vi "CheezyAcos.vi"(1 "arg":dbl) -> (0 "acos(arg)":dbl)   [LabVIEW 2016]
uses:
  <userlib>/836-Libraries/Math/CheezyMath/MathConstantsNames.ctl
panel:
  out "Time to run":dbl
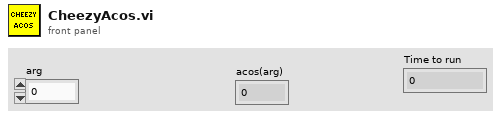
[diagram p1: front panel]
types:
  T1 = typedef "MathConstantsNames.ctl" = enum16{"sq2p1", "sq2m1", "p4", "p3", "p2", "p1", "p0", "q4", "q3", "q2", "q1", "q0", "PIO2"}
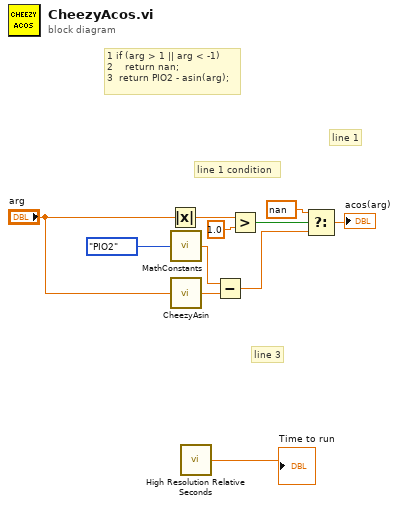
[diagram p0: block diagram]
diagram:
  # "line 3"
  # "line 1"
  # "line 1 condition"
  # "1 if (arg > 1 || arg < -1) \n2    return nan;\n3  return PIO2 - asin(arg);"
  n1 = Absolute Value(x="arg") -> (abs(x)=w11:dbl)
  n2 = call <userlib>:"MathConstants.vi"("Constant Name"=MathConstantsNames."PIO2") -> ("Constant Value"=w5:dbl)
  n3 = call <userlib>:"CheezyAsin.vi"("arg"="arg") -> ("asin(arg)"=w4:dbl)
  n4 = call <vilib>:"High Resolution Relative Seconds.vi"() -> ("relative seconds"=→"Time to run":dbl)
  n5 = Subtract(x=w5, y=w4) -> (x-y=w3:dbl)
  n6 = Greater?(x=w11, y=1.0) -> (0:w9:bool)
  n7 = Select(t=nan, s=w9, f=w3) -> (s? t:f=→"acos(arg)":dbl)
